vi "Plant_to_CH.vi"   [LabVIEW 2021, in "TimeBasedProd.lvlib"]
uses:
  TimeBasedProd.lvlib
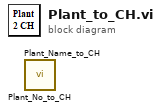
[diagram p0: block diagram]
diagram:
  n1 = call "Plant_No_to_CH.vi"() -> ()  [unwired: 10 in, 2 out]
  n2 = call "Plant_Name_to_CH.vi"() -> ()  [unwired: 8 in, 4 out]
